vi "DBC2Sheet.vi"(4 "进度数值":refnum<vi>, 5 "Slide输入":refnum<vi>, 6 "DBC树":refnum<vi>, 7 "ValueTable":refnum<vi>, 8 "file path (dialog if empty)":path) -> (0 "值表数组":string[][](array[string]), 1 "信号数":i32, 2 "数组":string[][](array[string]), 3 "报文数":i32)   [LabVIEW 2015]
uses:
  <vilib>/Utility/file.llb/Read Delimited Spreadsheet (string).vi
panel:
  out "Language":u32
  out "进度数值":string="0%"
  out "水平进度条":u8(slide) scale=0.0..100.0
  # "通叔提示您：程序正在玩命解析DBC文件，请稍后..."
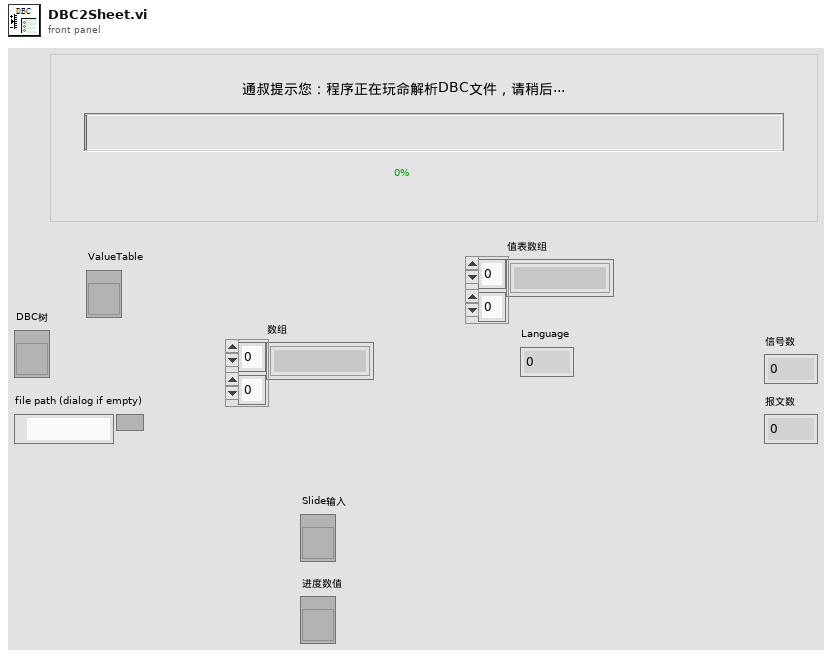
[diagram p1: front panel]
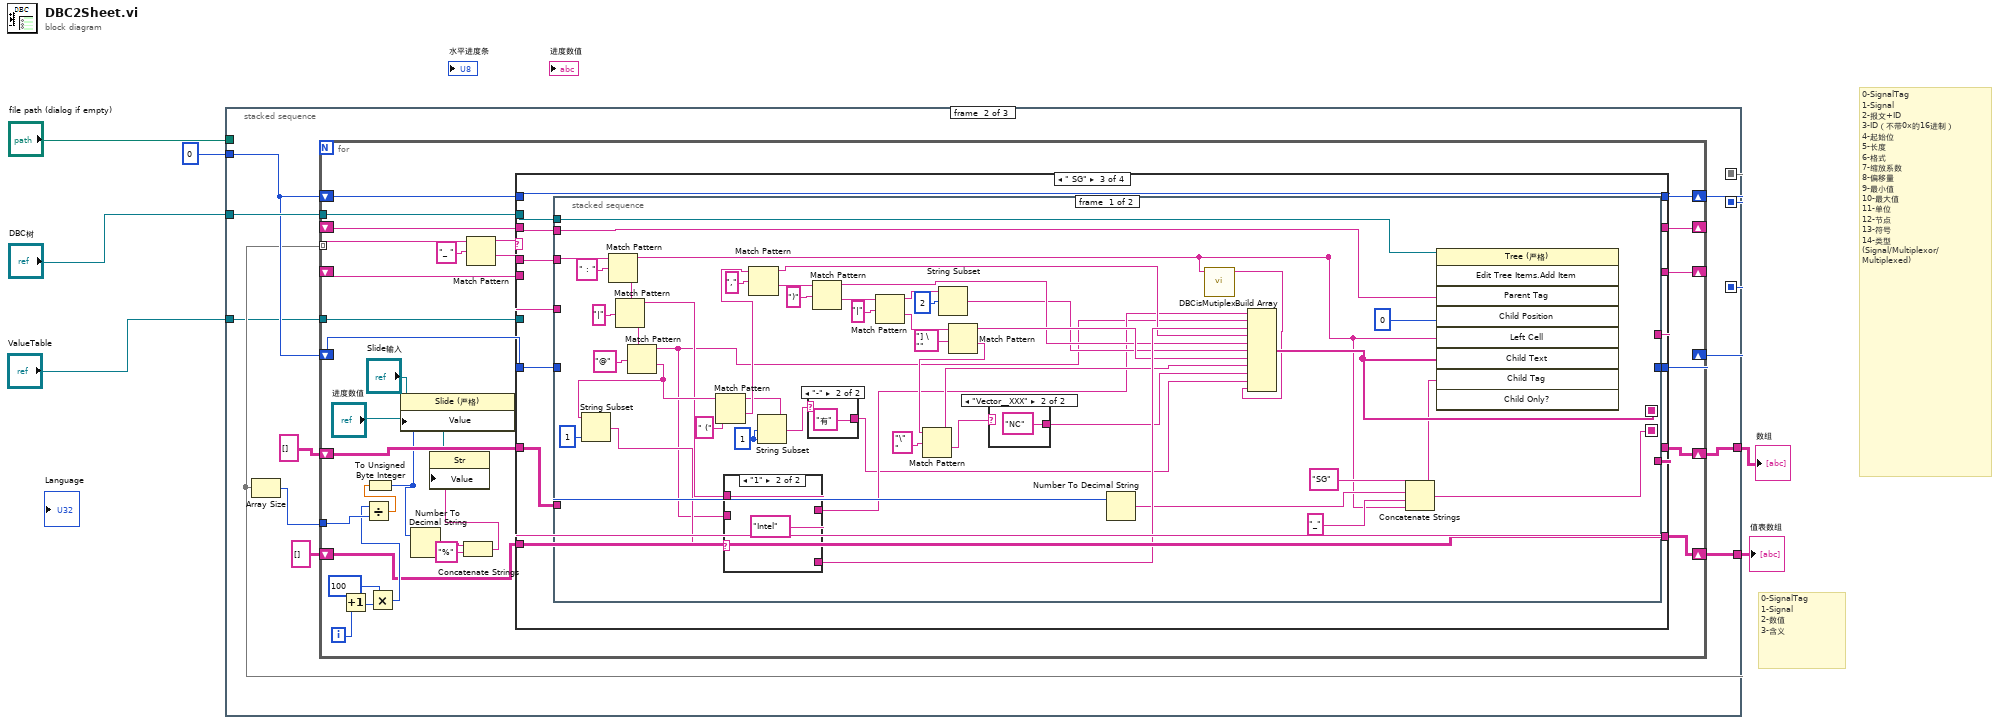
[diagram p0: block diagram]
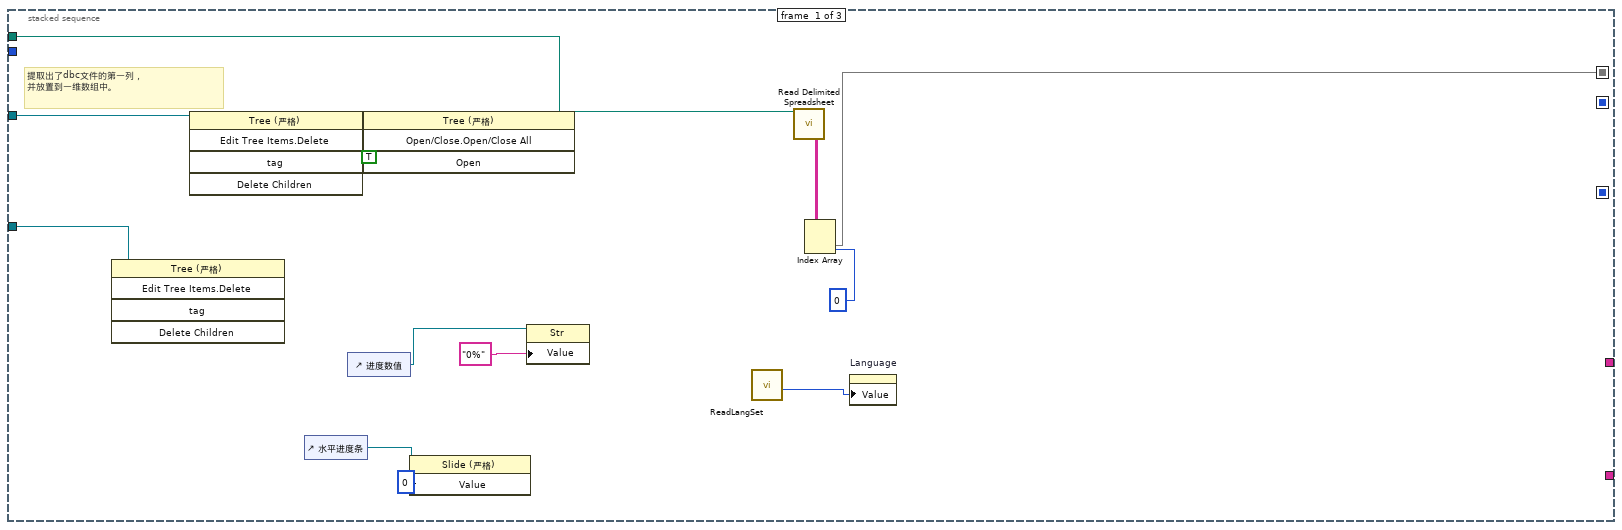
[diagram p2: hidden frame]
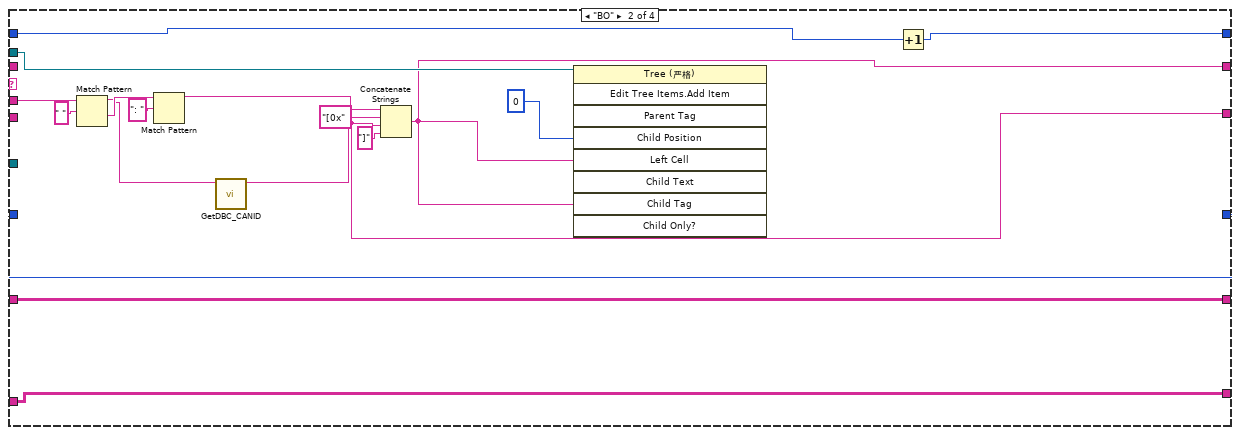
[diagram p4: hidden frame]
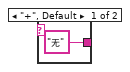
[diagram p5: hidden frame]
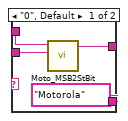
[diagram p7: hidden frame]
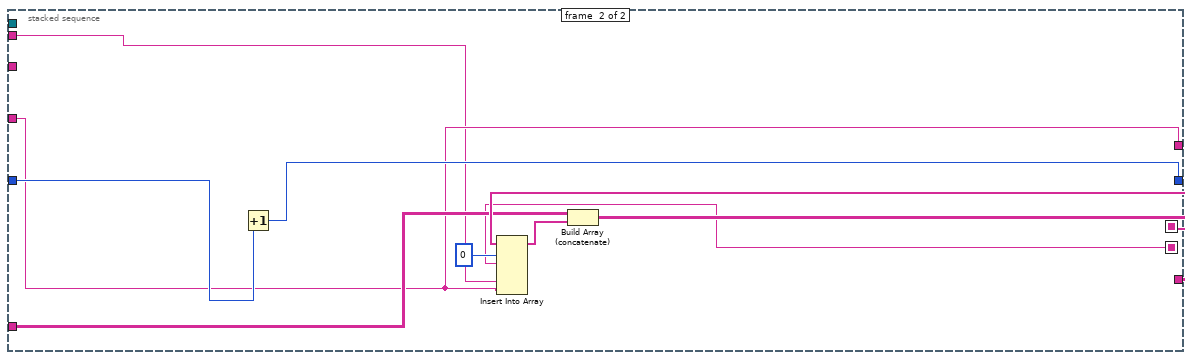
[diagram p8: hidden frame]
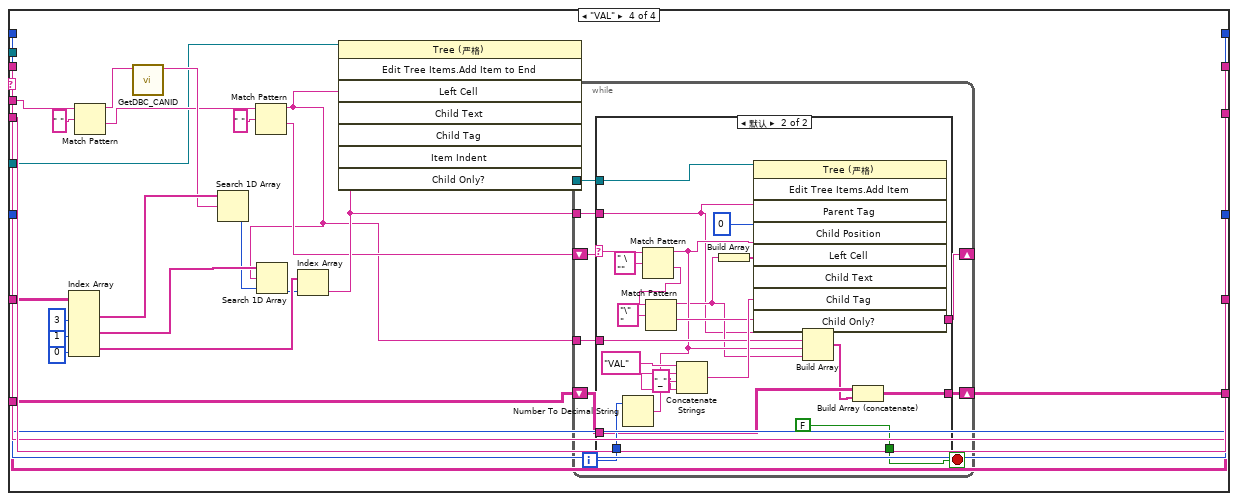
[diagram p9: hidden frame]
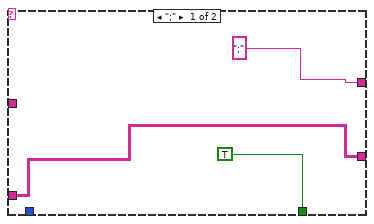
[diagram p10: hidden frame]
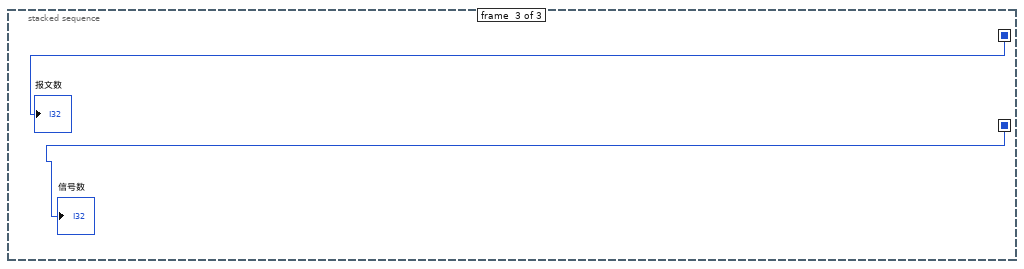
[diagram p11: hidden frame]
diagram:
  # "0-SignalTag\n1-Signal\n2-数值\n3-含义"
  # "0-SignalTag\n1-Signal\n2-报文+ID\n3-ID（不带0x的16进制）\n4-起始位\n5-长度\n6-格式\n7-缩放系数\n8-偏移量\n9-最小值\n10-最大值\n11-单位\n12-节点\n13-符号\n14-类型\n(Signal/Multiplexor/\nMultiplexed)"
  n1 = stacked-sequence {
    seq-local: [w16 _ _] -> [_ w24 _]
    seq-local: [_ w29 _] -> [_ _ w223]
    seq-local: [_ w27 _] -> [_ _ w224]
    tunnel: "file path (dialog if empty)" -> [w18 _ _]
    tunnel: "DBC树" -> [w13 w30 _]
    tunnel: 0 -> [_ w28 _]
    tunnel: [_ w26 _] -> w3
    tunnel: "ValueTable" -> [w8 w22 _]
    tunnel: [_ w20 _] -> w1
    frame #0 {
      # "提取出了dbc文件的第一列，\n并放置到一维数组中。"
      n2 = invoke on="调用节点" class="Tree (严格)" method="Edit Tree Items.Delete"(reference=w8) -> ()  [unwired: 4 in, 5 out]
      n3 = invoke on="调用节点" class="Tree (严格)" method="Edit Tree Items.Delete"(reference=w13) -> (reference out=w14:refnum<vi>)  [unwired: 4 in, 4 out]
      n4 = control-ref of="水平进度条"() -> (w10:refnum<vi>)
      n5 = control-ref of="进度数值"() -> (w12:refnum<vi>)
      n6 = invoke on="调用节点" class="Tree (严格)" method="Open/Close.Open/Close All"(reference=w14, "Open"=TRUE ("打开？")) -> ()  [unwired: 2 in, 4 out]
      n7 = property class="Slide (严格)"(reference=w10, "Value"=u8 0 ("值")) -> ()  [unwired: 1 in, 2 out]
      n8 = property class="Str"(reference=w12, "Value"="0%" ("值")) -> ()  [unwired: 1 in, 2 out]
      n9 = call "ReadLangSet.vi"() -> ("Language"=w7:u32)  [unwired: 11 in]
      n10 = call-poly <vilib>:"Read Delimited Spreadsheet.vi"("file path (dialog if empty)"=w18) -> ("all rows"=w17:string[][])  [unwired: 9 in, 5 out]
      n11 = Index Array(array=w17, index (col)=0 ("禁用的索引 (列)")) -> (element=w16:string[])  [unwired: 1 in]
      n12 = property on="Language" class="DigNum (严格)"("Value"=w7) -> ()  [unwired: 2 in, 2 out]
    }
    frame #1 {
      n13 = Array Size(array=w24) -> (size(s)=w23:i32)
      n14 = for {
        tunnel: w24 -> [w60] mode=indexing
        shift-right: [w59] -> _
        shift-left: _ -> [w58]
        tunnel: w30 -> [w54]
        shift-right: [w53] -> w29
        shift-left: w28 -> [w52]
        shift-right: [w50] -> w27
        shift-left: w28 -> [w51]
        shift-right: [w49] -> w26
        shift-left: string[][] [] -> [w48]
        shift-right: [w47] -> _
        shift-left: _ -> [w46]
        tunnel: w23 -> [w44]
        tunnel: w22 -> [w35]
        shift-right: [w33] -> w20
        shift-left: string[][] [] -> [w34]
        i -> [w45]
        n15 = Increment(x=w45) -> (x+1=w38:i32)
        n16 = Multiply(x=100, y=w38) -> (x*y=w36:i32)
        n17 = Divide(x=w36, y=w44) -> (x/y=w43:dbl)
        n18 = To Unsigned Byte Integer(number=w43) -> (unsigned 8bit integer=w42:u8)
        n19 = property class="Slide (严格)"(reference="Slide输入", "Value"=w42) -> ()  [unwired: 1 in, 2 out]
        n20 = Number To Decimal String(number=w42) -> (decimal integer string=w41:string)  [unwired: 1 in]
        n21 = Concatenate Strings(w41, "%" ("字符串")) -> (w39:string)
        n22 = property class="Str"(reference="进度数值", "Value"=w39) -> ()  [unwired: 1 in, 2 out]
        n23 = Match Pattern(string=w60, regular expression="_ " ("正则表达式")) -> (before substring=w56:string, after substring=w55:string)  [unwired: 1 in, 2 out]
        n24 = case shown="\" SG\"" w56 {
          tunnel: w55 -> [_ w83 w94 w184]
          tunnel: [w66 w68 w93 w188] -> w59
          tunnel: w58 -> [w66 _ w93 w188]
          tunnel: w54 -> [_ w69 w92 _]
          tunnel: w52 -> [w65 w76 w91 w187]
          tunnel: [w65 w75 w91 w187] -> w53
          tunnel: w51 -> [w64 w74 w90 w186]
          tunnel: [w64 w74 w89 w186] -> w50
          tunnel: [w63 w73 w88 w182] -> w49
          tunnel: w48 -> [w63 w73 w87 w182]
          tunnel: [w62 w71 w85 w189] -> w47
          tunnel: w46 -> [w62 _ w86 w189]
          tunnel: w35 -> [_ _ _ w170]
          tunnel: w34 -> [w61 w70 w84 w164]
          tunnel: [w61 w70 w84 w166] -> w33
          frame Default {
          }
          frame "BO" {
            n25 = Match Pattern(string=w83, regular expression=" " ("正则表达式")) -> (before substring=w79:string, after substring=w81:string)  [unwired: 1 in, 2 out]
            n26 = Match Pattern(string=w81, regular expression=": " ("正则表达式")) -> (before substring=w72:string)  [unwired: 1 in, 3 out]
            n27 = call "GetDBC_CANID.vi"("String"=w79) -> ("字符串"=w71:string)  [unwired: 10 in]
            n28 = Concatenate Strings(w72, "[0x" ("字符串"), w71, "]" ("字符串")) -> (w68:string)
            n29 = invoke class="Tree (严格)" method="Edit Tree Items.Add Item"(reference=w69, "Child Position"=0 ("子项位置"), "Left Cell"=w68, "Child Tag"=w68) -> ()  [unwired: 5 in, 9 out]
            n30 = Increment(x=w76) -> (x+1=w75:i32)
          }
          frame " SG" {
            n31 = stacked-sequence {
              seq-local: [w96 _] -> [_ w153]
              seq-local: [w112 _] -> [_ w159]
              seq-local: [w109 _] -> [_ w154]
              tunnel: w94 -> [w142 _]
              tunnel: w93 -> [w113 w155]
              tunnel: w92 -> [w114 _]
              tunnel: w90 -> [w111 w163]
              tunnel: [_ w162] -> w89
              tunnel: [_ w158] -> w88
              tunnel: w87 -> [_ w157]
              tunnel: w86 -> [_ w156]
              tunnel: [_ w156] -> w85
              frame #0 {
                w100 = 1 ("长度（剩余）")
                n32 = Match Pattern(string=w142, regular expression=" : " ("正则表达式")) -> (before substring=w96:string, after substring=w140:string)  [unwired: 1 in, 2 out]
                n33 = Match Pattern(string=w140, regular expression="|" ("正则表达式")) -> (before substring=w105:string, after substring=w138:string)  [unwired: 1 in, 2 out]
                n34 = Match Pattern(string=w138, regular expression="@" ("正则表达式")) -> (before substring=w103:string, after substring=w108:string)  [unwired: 1 in, 2 out]
                n35 = String Subset(string=w108, length (rest)=1 ("长度（剩余）")) -> (substring=w106:string)  [unwired: 1 in]
                n36 = Match Pattern(string=w108, regular expression=" (" ("正则表达式")) -> (before substring=w99:string, after substring=w125:string)  [unwired: 1 in, 2 out]
                n37 = case shown="\"1\"" w106 {
                  tunnel: ["Motorola" "Intel"] -> w135
                  tunnel: w105 -> [w149 w151]
                  tunnel: [w148 w151] -> w104
                  tunnel: w103 -> [w147 _]
                  frame "0", Default {
                    n38 = call "Moto_MSB2StBit.vi"("长度"=w147, "MSB"=w149) -> ("起始位"=w148:string)  [unwired: 9 in]
                  }
                  frame "1" {
                  }
                }
                n39 = Match Pattern(string=w125, regular expression="," ("正则表达式")) -> (before substring=w124:string, after substring=w123:string)  [unwired: 1 in, 2 out]
                n40 = String Subset(string=w99, offset (0)=w100, length (rest)=w100) -> (substring=w98:string)
                n41 = case shown="\"-\"" w98 {
                  tunnel: ["无" "有"] -> w97
                  frame "+", Default {
                  }
                  frame "-" {
                  }
                }
                n42 = Match Pattern(string=w123, regular expression=")" ("正则表达式")) -> (before substring=w122:string, after substring=w121:string)  [unwired: 1 in, 2 out]
                n43 = Match Pattern(string=w121, regular expression="|" ("正则表达式")) -> (before substring=w120:string, after substring=w131:string)  [unwired: 1 in, 2 out]
                n44 = String Subset(string=w120, offset (0)=2 ("偏移量(0)")) -> (substring=w119:string)  [unwired: 1 in]
                n45 = Match Pattern(string=w131, regular expression="] \"" ("正则表达式")) -> (before substring=w129:string, after substring=w128:string)  [unwired: 1 in, 2 out]
                n46 = Match Pattern(string=w128, regular expression="\" " ("正则表达式")) -> (before substring=w126:string, after substring=w116:string)  [unwired: 1 in, 2 out]
                n47 = case shown="\"Vector__XXX\"" w116 {
                  selector: w116 -> [w145 _]
                  tunnel: [w145 "NC"] -> w117
                  frame Default {
                  }
                  frame "Vector__XXX" {
                  }
                }
                n48 = Number To Decimal String(number=w111) -> (decimal integer string=w110:string)  [unwired: 1 in]
                n49 = call "DBCisMutiplex.vi"("Sg"=w96) -> ("Style10"=w95:string)  [unwired: 10 in]
                n50 = Build Array(w104, w103, w135, w124, w122, w119, w129, w126, w117, w97, w95) -> (w112:string[])
                n51 = Concatenate Strings("SG" ("字符串"), w110, "_" ("字符串"), w96) -> (w109:string)
                n52 = invoke class="Tree (严格)" method="Edit Tree Items.Add Item"(reference=w114, "Parent Tag"=w113, "Child Position"=0 ("子项位置"), "Left Cell"=w96, "Child Text"=w112, "Child Tag"=w109) -> ()  [unwired: 3 in, 9 out]
              }
              frame #1 {
                n53 = Increment(x=w163) -> (x+1=w162:i32)
                n54 = Insert Into Array(array=w159, index=0 ("索引"), new element #1=w154, new element #2=w153, new element #3=w155, new element #4=w156) -> (w160:string[])
                n55 = Build Array (concatenate)(w157, w160) -> (w158:string[][])
              }
            }
          }
          frame "VAL" {
            n56 = Index Array(array=w182, index (col) #1=3 ("禁用的索引 (列)"), index (col) #2=1 ("索引 (列)"), index (col) #3=0 ("索引 (列)")) -> (element #1=w180:string[], element #2=w177:string[], element #3=w172:string[])  [unwired: 3 in]
            n57 = Match Pattern(string=w184, regular expression=" " ("正则表达式")) -> (before substring=w183:string, after substring=w175:string)  [unwired: 1 in, 2 out]
            n58 = call "GetDBC_CANID.vi"("String"=w183) -> ("字符串"=w179:string)  [unwired: 10 in]
            n59 = Search 1D Array(1D array=w180, element=w179) -> (index of element=w174:i32)  [unwired: 1 in]
            n60 = Match Pattern(string=w175, regular expression=" " ("正则表达式")) -> (before substring=w165:string, after substring=w168:string)  [unwired: 1 in, 2 out]
            n61 = Search 1D Array(1D array=w177, element=w165, start index (0)=w174) -> (index of element=w171:i32)
            n62 = Index Array(array=w172, index=w171) -> (element=w169:string)
            n63 = invoke class="Tree (严格)" method="Edit Tree Items.Add Item to End"(reference=w170, "Left Cell"=w165, "Child Tag"=w169) -> (reference out=w167:refnum<vi>)  [unwired: 5 in, 7 out]
            n64 = while {
              tunnel: w169 -> [w198]
              shift-right: [w193] -> _
              shift-left: w168 -> [w197]
              tunnel: w167 -> [w194]
              tunnel: w165 -> [w191]
              shift-right: [w192] -> w166
              shift-left: w164 -> [w190]
              i -> [w195]
              stop <- w196 stop-if-true
              n65 = case shown="默认" w197 {
                selector: w197 -> [_ w222]
                tunnel: w198 -> [_ w202]
                tunnel: [TRUE FALSE] -> w196
                tunnel: w195 -> [_ w218]
                tunnel: w194 -> [_ w214]
                tunnel: [";" w210] -> w193
                tunnel: w190 -> [w199 w209]
                tunnel: [w199 w208] -> w192
                tunnel: w191 -> [_ w206]
                frame ";" {
                }
                frame Default {
                  n66 = Number To Decimal String(number=w218) -> (decimal integer string=w217:string)  [unwired: 1 in]
                  n67 = Match Pattern(string=w222, regular expression=" \"" ("正则表达式")) -> (before substring=w205:string, after substring=w216:string)  [unwired: 1 in, 2 out]
                  n68 = Match Pattern(string=w216, regular expression="\" " ("正则表达式")) -> (before substring=w204:string, after substring=w210:string)  [unwired: 1 in, 2 out]
                  n69 = Concatenate Strings("VAL" ("字符串"), w217, "_" ("字符串"), w205) -> (w213:string)
                  n70 = Build Array(w204) -> (w211:string[])
                  n71 = invoke class="Tree (严格)" method="Edit Tree Items.Add Item"(reference=w214, "Parent Tag"=w202, "Child Position"=0 ("子项位置"), "Left Cell"=w205, "Child Text"=w211, "Child Tag"=w213) -> ()  [unwired: 3 in, 9 out]
                  n72 = Build Array(w202, w206, w205, w204) -> (w203:string[])
                  n73 = Build Array (concatenate)(w209, w203) -> (w208:string[][])
                }
              }
            }
          }
        }
      }
    }
    frame #2 {
      "信号数" <- w224
      "报文数" <- w223
    }
  }
  "数组" <- w3
  "值表数组" <- w1
